vi "Initialize Instrument.vi"(8 "error in (no error)":errorcluster, 10 "Reset":bool, 11 "Tektronix TDS 200 1000 2000 in":refnum<class "Tektronix TDS 200 1000 2000.lvclass">) -> (0 "error out":errorcluster, 3 "Tektronix TDS 200 1000 2000 out":refnum<class "Tektronix TDS 200 1000 2000.lvclass">)   [LabVIEW 2020, in "Tektronix TDS 200 1000 2000.lvclass"]
uses:
  Tektronix TDS 200 1000 2000.lvclass
  C:/Sandbox/RF Bench/Source Code/WiSpry Test Framework/Instruments/Instrument.lvclass
  Instrument.lvclass/Instrument.ctl
  Instrument.lvclass
  <instrlib>/Tektronix TDS 200 1000 2000 Series/Tektronix TDS 200 1000 2000 Series.lvlib
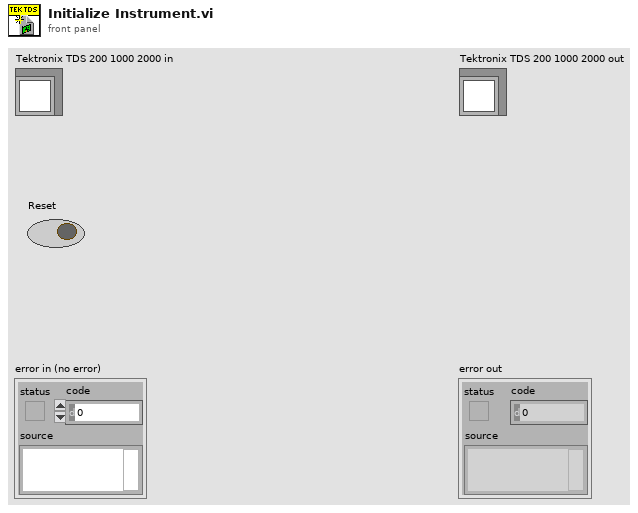
[diagram p1: front panel]
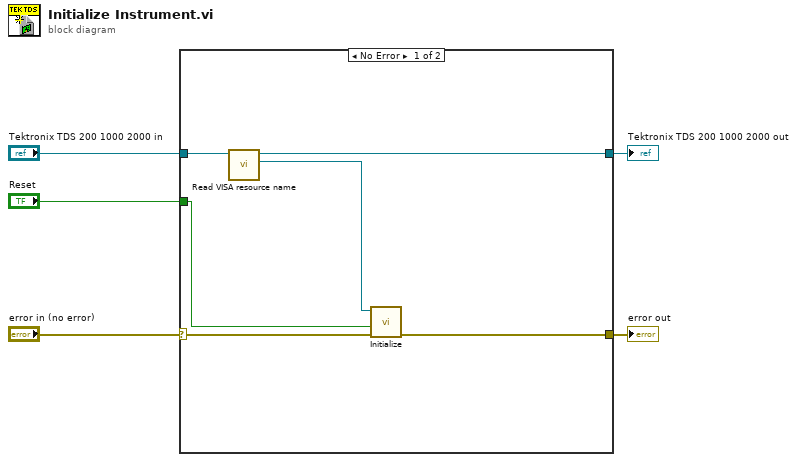
[diagram p0: block diagram]
diagram:
  n1 = case shown="No Error" "error in (no error)" {
    selector: "error in (no error)" -> [w9 w13]
    tunnel: [w8 w13] -> w2
    tunnel: [w10 w12] -> w3
    tunnel: "Tektronix TDS 200 1000 2000 in" -> [w11 w12]
    tunnel: "Reset" -> [w6 _]
    frame No Error {
      n2 = call "Read VISA resource name.vi"("Instrument in"=w11) -> ("VISA resource name"=w7:refnum<visa-resource-name>, "Instrument out"=w10:refnum<class "Tektronix TDS 200 1000 2000.lvclass">)  [unwired: 9 in]
      n3 = call <instrlib>:"Initialize.vi"("error in (no error)"=w9, "Reset? (T: Yes)"=w6, "VISA resource name"=w7) -> ("error out"=w8:errorcluster)  [unwired: 7 in, 1 out]
    }
    frame Error {
    }
  }
  "error out" <- w2
  "Tektronix TDS 200 1000 2000 out" <- w3
